vi "Water Tank Level Indicator.vi"() -> ()   [LabVIEW 2022 SP3]
panel:
  in  "duration (msec)":u32
  in  "Minimum":dbl(slide) scale=0.0..100.0
  out "Current Water Level":dbl
  in  "stop":bool
  out "Maximum":bool
  out "Minimum":bool
  out "Tank":dbl(slide) scale=0.0..100.0
  in  "Maximum":dbl(slide) scale=0.0..100.0
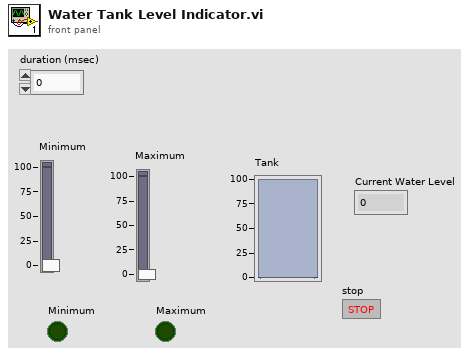
[diagram p1: front panel]
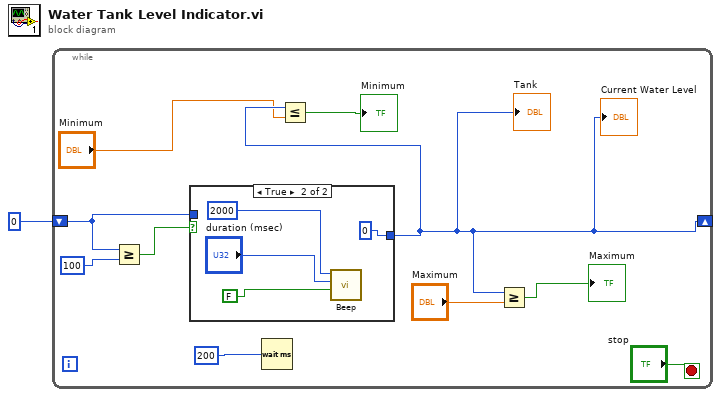
[diagram p0: block diagram]
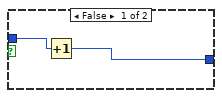
[diagram p2: hidden frame]
diagram:
  n1 = while {
    shift-right: [w3] -> _
    shift-left: 0 -> [w4]
    stop <- "stop" stop-if-true
    n2 = Greater Or Equal?(x=w4, y=100) -> (x >= y?=w5:bool)
    n3 = case shown="True" w5 {
      tunnel: w4 -> [w13 _]
      tunnel: [w12 0] -> w3
      frame False {
        n4 = Increment(x=w13) -> (x+1=w12:i32)
      }
      frame True {
        n5 = call <vilib>:"Beep.vi"("use system alert? (T)"=FALSE, "duration (msec)"="duration (msec)", "frequency (Hz)"=u32 2000) -> ()  [unwired: 9 in]
      }
    }
    "Tank" <- w3
    "Current Water Level" <- w3
    n6 = Wait (ms)(milliseconds to wait=u32 200 ("millisecond timer value")) -> ()  [unwired: 1 out]
    n7 = Less Or Equal?(x=w3, y="Minimum") -> (x <= y?=→"Minimum":bool)
    n8 = Greater Or Equal?(x=w3, y="Maximum") -> (x >= y?=→"Maximum":bool)
  }
